vi "Управление нагревом.vi"(0 "Температура arr":refnum<vi>, 5 "Stop":refnum<vi>, 6 "inpet_lable":string[](array[string])=["Кернодержатель", "Корпус", "Термошкаф", "Камера насосов", "Ш 1", "Ш 2", "Ш 3", "Ш 4"], 8 "Вызов":refnum<vi>, 9 "Термошкаф":refnum<vi>) -> ()   [LabVIEW 2018]
uses:
  <vilib>/addons/control/pid/NI_PID_pid.lvlib
  <vilib>/addons/control/pid/pid.llb/PID (DBL Array).vi
panel:
  in  "Boolean":bool
  in  "PID gains":T1(array[cluster])=[{"Kc"=30.0, "Ti, min"=20.0, "Td, min"=0.0}, {"Kc"=60.0, "Ti, min"=10.0, "Td, min"=0.0}, {"Kc"=90.0, "Ti, min"=15.0, "Td, min"=0.0}, {"Kc"=90.0, "Ti, min"=5.0, "Td, min"=0.0}, {"Kc"=90.0, "Ti, min"=5.0, "Td, min"=0.0}, {"Kc"=90.0, "Ti, min"=15.0, "Td, min"=0.0}, {"Kc"=90.0, "Ti, min"=15.0, "Td, min"=0.0}, {"Kc"=90.0, "Ti, min"=15.0, "Td, min"=0.0}, {"Kc"=90.0, "Ti, min"=15.0, "Td, min"=0.0}] {"Td, min" format="%.3f"; "Ti, min" format="%.3f"; "Kc" format="%.3f"}
  out "DAC":u16[](array[numeric])
  in  "Tarr2":dbl[](array[numeric])
  in  "Tarr1":dbl[](array[numeric])
  in  "on/off_control_1":bool[](array[boolean])=[FALSE, FALSE, FALSE, FALSE, FALSE, FALSE, FALSE, FALSE]
  in  "sp_control_1":dbl[](array[numeric])=[20.0, 20.0, 20.0, 20.0, 20.0, 20.0, 20.0, 20.0] min=20.0 max=150.0 step=0.1 format="%#.1f"
  out "pv_indic_1":dbl[](array[numeric])=[20.0, 20.0, 20.0, 20.0, 20.0, 20.0, 20.0, 20.0] min=20.0 max=150.0 step=0.1 format="%#.1f"
  in  "Закрыть":bool
  out "label_indic_1":string[](array[string])=["Кернодержатель 1", "Кернодержатель 2", "Кернодержатель 3", "Кернодержатель 4", "Кернодержатель 5", "Кернодержатель 6", "Кернодержатель 7", "Кернодержатель 8"]
  # "Задание температуры"
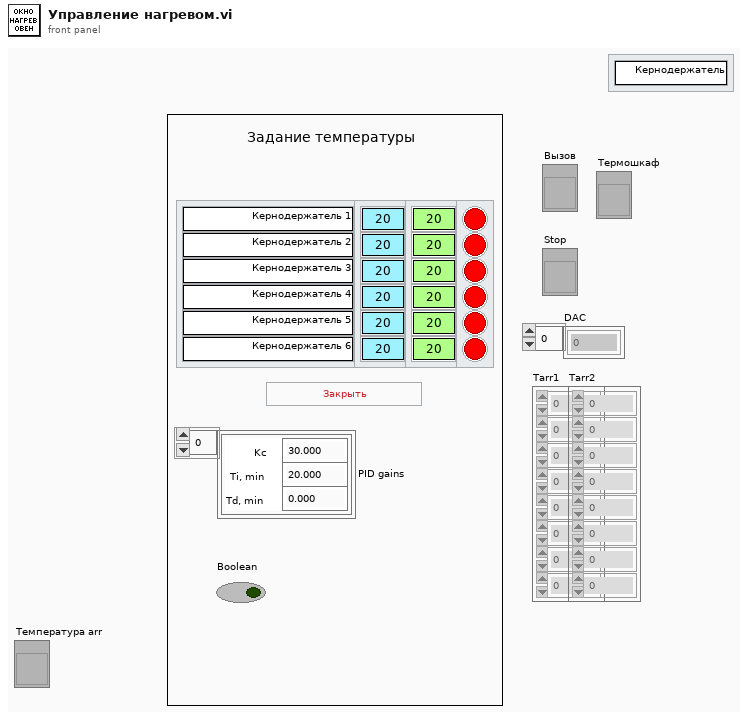
[diagram p1: front panel]
types:
  T1 = cluster{"Kc":dbl, "Ti, min":dbl, "Td, min":dbl}[]
  T2 = enum16{"big-endian, network order", "native, host order", "little-endian"}
  T3 = enum16{"open", "replace", "create", "open or create", "replace or create", "replace or create with confirmation"}
  T4 = cluster{"PID gains":cluster{"Kc":dbl, "Ti, min":dbl, "Td, min":dbl}[]}[]
  T5 = cluster{"PID gains":cluster{"Kc":dbl, "Ti, min":dbl, "Td, min":dbl}[]}
  T6 = enum32{"invalid app kind", "Development System", "Run Time System", "Student Edition", "Embedded LabVIEW", "Evaluation", "Custom"}
  T7 = enum32{"Invalid", "Standard", "Closed", "Hidden", "Minimized", "Maximized"}
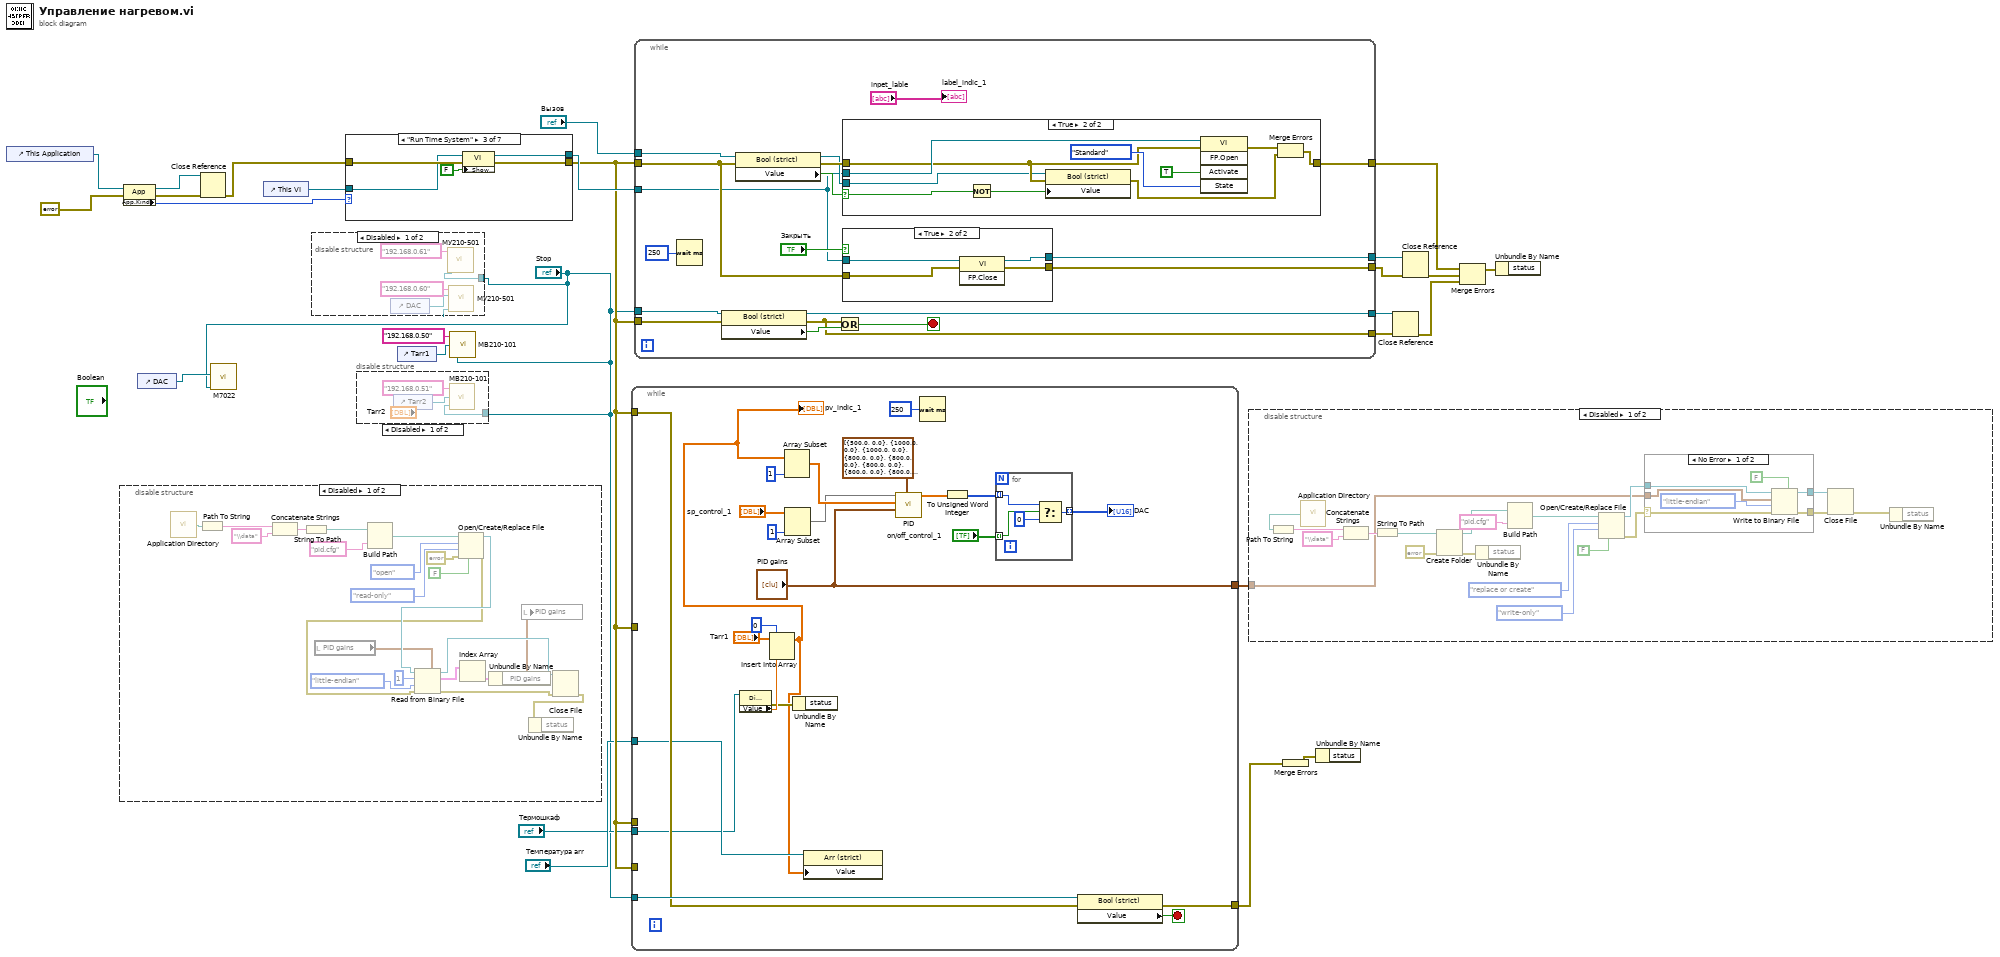
[diagram p0: block diagram]
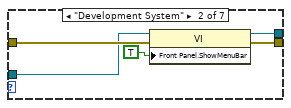
[diagram p8: hidden frame]
diagram:
  n1 = control-ref of="This Application"() -> (w24:refnum<vi>)
  n2 = disable-structure shown="Disabled" {
    frame Disabled {
      n3 = call <vilib>:"Application Directory.vi"() -> ("Application Directory"=w45:path)
      n4 = Path To String(path=w45) -> (string=w46:string)
      n5 = Concatenate Strings(w46, "\\data" ("string")) -> (w47:string)
      n6 = String To Path(string=w47) -> (path=w49:path)
      n7 = local read "PID gains"() -> (w34:T1)
      n8 = Build Path(base path=w49, name or relative path="pid.cfg") -> (appended path=w48:path)
      n9 = Open/Create/Replace File(file path (use dialog)=w48, error in=errorcluster {"status"=FALSE, "code"=0, "source"=""}, operation (0:open)=T3."open", access (0:read/write)=enum16{"read/write", "read-only", "write-only"}."read-only", disable buffering (F)=FALSE) -> (refnum out=w36:refnum<file>, error out=w35:errorcluster)  [unwired: 1 in, 1 out]
      n10 = Read from Binary File(5:w34, 8:w35, 9:T2."little-endian" ("byte order (0:big-endian, network order)"), 10:1 ("count (1)"), 11:w36) -> (0:w32:errorcluster, 2:w37:T4, 3:w31:refnum<file>)  [unwired: 1 in, 1 out]
      n11 = Index Array(array=w37) -> (element=w30:T5)  [unwired: 1 in]
      n12 = Unbundle By Name(w30) -> ("PID gains"=w29:T1)
      n13 = local write "PID gains"(w29) -> ()
      n14 = Close File(refnum=w31, error in=w32) -> (error out=w28:errorcluster)  [unwired: 1 out]
      n15 = Unbundle By Name(w28) -> ()  [unwired: 1 out]
    }
    frame Enabled {
    }
  }
  n16 = property class="App"(reference=w24, error in=errorcluster {"status"=FALSE, "code"=0, "source"=""} ("error in (no error)")) -> (reference out=w25:refnum<vi>, error out=w26:errorcluster, "App.Kind"=w22:T6)
  n17 = control-ref of="DAC"() -> (w2:refnum<vi>)
  n18 = Close Reference(reference=w25, error in (no error)=w26) -> (error out=w21:errorcluster)
  n19 = call "М7022.vi"("stop"="Stop", "регистры"=w2) -> ()  [unwired: 10 in]
  n20 = control-ref of="This VI"() -> (w27:refnum<vi>)
  n21 = disable-structure shown="Disabled" {
    disable-tunnel: "Stop" -> [w50 _]
    frame Disabled {
      n22 = control-ref of="DAC"() -> (w53:refnum<vi>)
      n23 = call "МУ210-501.vi"("stop"=w50, "IP Address"="192.168.0.61") -> ("регистры"=w51:refnum<vi>)  [unwired: 9 in]
      n24 = call "МУ210-501.vi"("stop"=w50, "регистры"=w53, "IP Address"="192.168.0.60") -> ()  [unwired: 9 in]
    }
    frame Enabled {
    }
  }
  n25 = case shown="\"Run Time System\"" w22 {
    tunnel: w21 -> [w55 w61 w65 w68 w69 w71 w73]
    tunnel: w27 -> [w56 w60 w64 w67 w70 w72 w74]
    tunnel: [w56 w58 w63 w67 w70 w72 w74] -> w19
    tunnel: [w55 w57 w62 w68 w69 w71 w73] -> w8
    frame "invalid app kind", Default {
    }
    frame "Development System" {
      n26 = property class="VI"(reference=w60, error in=w61, "Front Panel.ShowMenuBar"=TRUE ("Front Panel Window:Show Menu Bar")) -> (reference out=w58:refnum<vi>, error out=w57:errorcluster)
    }
    frame "Run Time System" {
      n27 = property class="VI"(reference=w64, error in=w65, "Front Panel.ShowMenuBar"=FALSE ("Front Panel Window:Show Menu Bar")) -> (reference out=w63:refnum<vi>, error out=w62:errorcluster)
    }
    frame "Student Edition" {
    }
    frame "Embedded LabVIEW" {
    }
    frame "Evaluation" {
    }
    frame "Custom" {
    }
  }
  n28 = disable-structure shown="Disabled" {
    disable-tunnel: "Stop" -> [w75 _]
    frame Disabled {
      n29 = control-ref of="Tarr2"() -> (w76:refnum<vi>)
      n30 = call "МВ210-101.vi"("Stop"=w75, "Tarr"=w76, "IP"="192.168.0.51") -> ()  [unwired: 1 in]
    }
    frame Enabled {
    }
  }
  n31 = control-ref of="Tarr1"() -> (w6:refnum<vi>)
  n32 = call "МВ210-101.vi"("Stop"="Stop", "Tarr"=w6, "IP"="192.168.0.50") -> ()  [unwired: 1 in]
  n33 = while {
    tunnel: w8 -> [w96]
    tunnel: "Stop" -> [w99]
    tunnel: [w98] -> w9
    tunnel: w8 -> [_]
    tunnel: w8 -> [_]
    tunnel: w8 -> [_]
    tunnel: ["PID gains"] -> w5
    tunnel: "Температура arr" -> [w84]
    tunnel: "Термошкаф" -> [w81]
    stop <- w100 stop-if-true
    n34 = property class="DigNum (strict)"(reference=w81) -> (error out=w79:errorcluster, "Value"=w80:dbl)  [unwired: 1 in, 1 out]
    n35 = Insert Into Array(array="Tarr1", index=0, new element=w80) -> (w78:dbl[])
    "pv_indic_1" <- w78
    n36 = Array Subset(array=w78, length=1) -> (w94:dbl[])  [unwired: 1 in]
    n37 = Array Subset(array="sp_control_1", length=1) -> (w91:dbl[])  [unwired: 1 in]
    n38 = Unbundle By Name(w79) -> ()  [unwired: 1 out]
    n39 = property class="Arr (strict)"(reference=w84, "Value"=w78) -> ()  [unwired: 1 in, 2 out]
    n40 = call-poly <vilib>:"PID.vi"("output range"=cluster{"output high":dbl, "output low":dbl}[] [{"output high"=500.0, "output low"=0.0}, {"output high"=1000.0, "output low"=0.0}, {"output high"=1000.0, "output low"=0.0}, {"output high"=800.0, "output low"=0.0}, {"output high"=800.0, "output low"=0.0}, {"output high"=800.0, "output low"=0.0}, {"output high"=800.0, "output low"=0.0}, {"output high"=800.0, "output low"=0.0}], "PID gains"="PID gains", "process variable"=w94, "setpoint"=w91) -> ("output"=w89:dbl[])  [unwired: 6 in, 1 out]
    n41 = Wait (ms)(milliseconds to wait=u32 250) -> ()  [unwired: 1 out]
    n42 = To Unsigned Word Integer(number=w89) -> (unsigned 16bit integer=w88:u16[])
    n43 = for {
      tunnel: w88 -> [w103] mode=indexing
      tunnel: "on/off_control_1" -> [w104] mode=indexing
      tunnel: [w101] -> w86 mode=indexing
      n44 = Select(t=w103, s=w104, f=u16 0) -> (s? t:f=w101:u16)
    }
    "DAC" <- w86
    n45 = property class="Bool (strict)"(reference=w99, error in=w96) -> (error out=w98:errorcluster, "Value"=w100:bool)  [unwired: 1 out]
  }
  n46 = while {
    tunnel: w19 -> [w107]
    tunnel: w8 -> [w111]
    tunnel: [w119] -> w15
    tunnel: [w120] -> w14
    tunnel: "Stop" -> [w118]
    tunnel: w8 -> [w106]
    tunnel: [w115] -> w13
    tunnel: [w114] -> w12
    tunnel: [w113] -> w11
    tunnel: "Вызов" -> [w112]
    stop <- w116 stop-if-true
    n47 = Wait (ms)(milliseconds to wait=u32 250) -> ()  [unwired: 1 out]
    n48 = property class="Bool (strict)"(reference=w118, error in=w106) -> (reference out=w115:refnum<vi>, error out=w114:errorcluster, "Value"=w117:bool)
    n49 = property class="Bool (strict)"(reference=w112, error in=w111) -> (reference out=w108:refnum<vi>, error out=w109:errorcluster, "Value"=w110:bool)
    n50 = Or(x=w114, y=w117) -> (x .or. y?=w116:bool)
    n51 = case shown="True" w110 {
      selector: w110 -> [_ w128]
      tunnel: [w123 w124] -> w113
      tunnel: w107 -> [_ w131]
      tunnel: w109 -> [w123 w130]
      tunnel: w108 -> [_ w129]
      frame False {
      }
      frame True {
        n52 = Not(x=w128) -> (.not. x?=w127:bool)
        n53 = property class="Bool (strict)"(reference=w129, error in=w130, "Value"=w127) -> (error out=w126:errorcluster)  [unwired: 1 out]
        n54 = invoke class="VI" method="FP.Open"(reference=w131, error in=w130, "Activate"=TRUE ("Activate?"), "State"=T7."Standard") -> (error out=w125:errorcluster)  [unwired: 1 in, 4 out]
        n55 = Merge Errors(w125, w126) -> (w124:errorcluster)
      }
    }
    n56 = case shown="True" "Закрыть" {
      tunnel: w107 -> [w134 w139]
      tunnel: w111 -> [w135 w138]
      tunnel: [w135 w137] -> w119
      tunnel: [w134 w136] -> w120
      frame False {
      }
      frame True {
        n57 = invoke class="VI" method="FP.Close"(reference=w139, error in=w138) -> (reference out=w136:refnum<vi>, error out=w137:errorcluster)  [unwired: 1 in, 1 out]
      }
    }
    "label_indic_1" <- "inpet_lable"
  }
  n58 = disable-structure shown="Disabled" {
    disable-tunnel: w5 -> [w141 _]
    frame Disabled {
      n59 = call <vilib>:"Application Directory.vi"() -> ("Application Directory"=w156:path)
      n60 = Path To String(path=w156) -> (string=w155:string)
      n61 = Concatenate Strings(w155, "\\data" ("string")) -> (w152:string)
      n62 = String To Path(string=w152) -> (path=w151:path)
      n63 = Create Folder(path (use dialog)=w151, error in=errorcluster {"status"=FALSE, "code"=0, "source"=""}) -> (created path=w145:path, error out=w143:errorcluster)  [unwired: 1 in, 1 out]
      n64 = Unbundle By Name(w143) -> ()  [unwired: 1 out]
      n65 = Build Path(base path=w145, name or relative path="pid.cfg") -> (appended path=w149:path)
      n66 = Open/Create/Replace File(file path (use dialog)=w149, operation (0:open)=T3."replace or create", access (0:read/write)=enum16{"read/write", "read-only", "write-only"}."write-only", disable buffering (F)=FALSE) -> (refnum out=w157:refnum<file>, error out=w158:errorcluster)  [unwired: 2 in, 1 out]
      n67 = case shown="No Error" w158 {
        selector: w158 -> [w163 w167]
        tunnel: w157 -> [w165 w166]
        tunnel: [w162 w167] -> w154
        tunnel: [w161 w166] -> w153
        tunnel: w141 -> [w159 _]
        frame No Error {
          n68 = Write to Binary File(file (use dialog)=w165, data=w159, error in=w163, 5:FALSE ("prepend array or string size? (T)"), 9:T2."little-endian" ("byte order (0:big-endian, network order)")) -> (refnum out=w161:refnum<file>, error out=w162:errorcluster)  [unwired: 1 in, 1 out]
        }
        frame Error {
        }
      }
      n69 = Close File(refnum=w153, error in=w154) -> (error out=w140:errorcluster)  [unwired: 1 out]
      n70 = Unbundle By Name(w140) -> ()  [unwired: 1 out]
    }
    frame Enabled {
    }
  }
  n71 = Merge Errors(w9) -> (w10:errorcluster)
  n72 = Unbundle By Name(w10) -> ()  [unwired: 1 out]
  n73 = Close Reference(reference=w13, error in (no error)=w12) -> (error out=w17:errorcluster)
  n74 = Close Reference(reference=w14, error in (no error)=w15) -> (error out=w18:errorcluster)
  n75 = Merge Errors(w11, w18, w17) -> (w16:errorcluster)
  n76 = Unbundle By Name(w16) -> ()  [unwired: 1 out]
